vi "niFpga wdp fft pfft 8.vi"(6 "enable":bool, 11 "data in":T2(array[cluster])=[{"data re"=0.0, "data im"=0.0}, {"data re"=0.0, "data im"=0.0}, {"data re"=0.0, "data im"=0.0}, {"data re"=0.0, "data im"=0.0}, {"data re"=0.0, "data im"=0.0}, {"data re"=0.0, "data im"=0.0}, {"data re"=0.0, "data im"=0.0}, {"data re"=0.0, "data im"=0.0}]) -> (3 "data out":T1(array[cluster]))   [LabVIEW 2017]
uses:
  <vilib>/rvi/FXPMathLib/FxpSub/XNode/nifxpmath_Sub.xnode
  <vilib>/rvi/FXPMathLib/FxpAdd/XNode/nifxpmath_Add.xnode
  <vilib>/rvi/FXPMathLib/FxpMul/XNode/nifxpmath_Multiplier.xnode
  <vilib>/rvi/FXPMathLib/sim/FxpSim.dll
types:
  T1 = cluster{"data re":fxp<+/-,8,1>, "data re":fxp<+/-,8,1>}[]
  T2 = cluster{"data re":fxp<+/-,8,1>, "data im":fxp<+/-,8,1>}[]
  T3 = cluster{"data re":fxp<+/-,8,1>, "data im":fxp<+/-,8,1>}
  T4 = cluster{"data re":fxp<+/-,8,1>, "data re":fxp<+/-,8,1>}
  T5 = cluster{"x*y":fxp<+/-,25,4>, "x*y":fxp<+/-,25,4>}
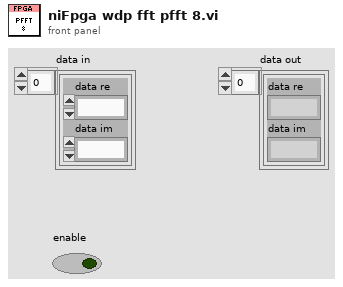
[diagram p1: front panel]
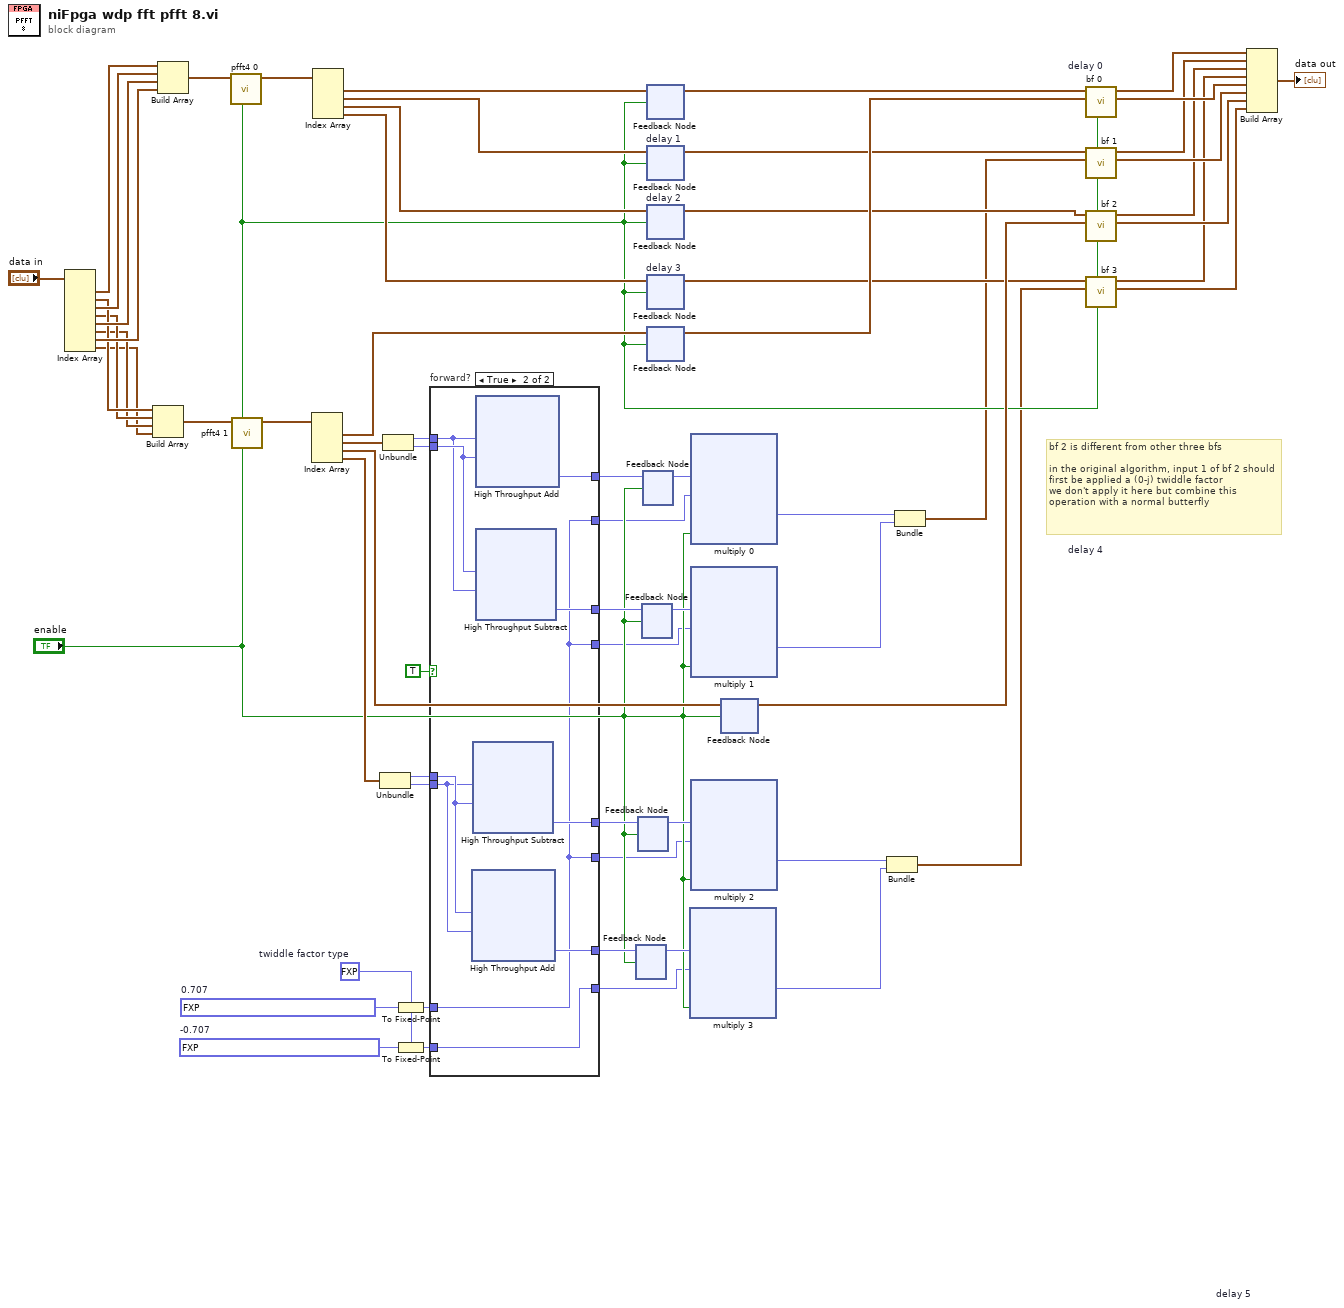
[diagram p0: block diagram]
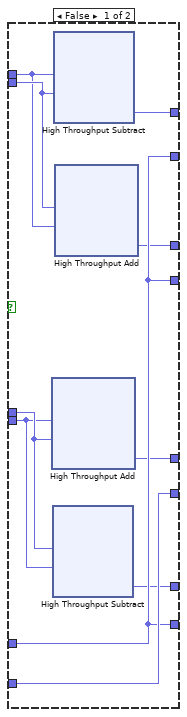
[diagram p2: hidden frame]
diagram:
  w36 = fxp<+/-,16,2> 0.0  # twiddle factor type
  w37 = fxp<+/-,32,2> -0.7071067811921239  # -0.707
  w38 = fxp<+/-,32,2> 0.7071067811921239  # 0.707
  # "bf 2 is different from other three bfs\n\nin the original algorithm, input 1 of bf 2 should first be applied a (0-j) twiddle factor\nwe don't apply it here but combine this operation with a normal butterfly"
  n1 = Index Array(array="data in") -> (element #1=w65:T3, element #2=w61:T3, element #3=w64:T3, element #4=w60:T3, element #5=w63:T3, element #6=w59:T3, element #7=w62:T3, element #8=w58:T3)  [unwired: 8 in]
  n2 = Build Array(w61, w60, w59, w58) -> (w32:T2)
  n3 = Build Array(w65, w64, w63, w62) -> (w34:T2)
  n4 = call "pfft4 0"("enable"="enable", "data in"=w34) -> ("data out"=w33:T1)  [unwired: 9 in]
  n5 = call "pfft4 1"("enable"="enable", "data in"=w32) -> ("data out"=w31:T1)  [unwired: 9 in]
  n6 = Index Array(array=w31) -> (element #1=w55:T4, element #2=w57:T4, element #3=w47:T4, element #4=w56:T4)  [unwired: 4 in]
  n7 = Index Array(array=w33) -> (element #1=w51:T4, element #2=w52:T4, element #3=w53:T4, element #4=w54:T4)  [unwired: 4 in]
  n8 = Unbundle(w56) -> ("data re"=w49:fxp<+/-,8,1>, "data re"=w48:fxp<+/-,8,1>)
  n9 = Unbundle(w57) -> ("data re"=w14:fxp<+/-,8,1>, "data re"=w50:fxp<+/-,8,1>)
  n10 = To Fixed-Point(fixed-point type=w36, number=w38) -> (fixed-point=w9:fxp<+/-,16,2>)
  n11 = To Fixed-Point(fixed-point type=w36, number=w37) -> (fixed-point=w7:fxp<+/-,16,2>)
  n12 = case "forward?" shown="True" TRUE {
    tunnel: w50 -> [w71 w85]
    tunnel: w49 -> [w68 w84]
    tunnel: w48 -> [w67 w83]
    tunnel: w14 -> [w70 w82]
    tunnel: [w73 w81] -> w46
    tunnel: [w72 w80] -> w44
    tunnel: [w69 w79] -> w42
    tunnel: [w66 w78] -> w40
    tunnel: [w74 w77] -> w12
    tunnel: [w74 w77] -> w11
    tunnel: [w75 w77] -> w10
    tunnel: w9 -> [w74 w77]
    tunnel: [w74 w76] -> w8
    tunnel: w7 -> [w75 w76]
    frame False {
      n13 = xnode ("High Throughput Add")("x"=w67, "y"=w68) -> ("x+y"=w69:fxp<+/-,9,2>)
      n14 = xnode "High Throughput Subtract"("x"=w68, "y"=w67) -> ("x-y"=w66:fxp<+/-,9,2>)
      n15 = xnode "High Throughput Subtract"("x"=w70, "y"=w71) -> ("x-y"=w73:fxp<+/-,9,2>)
      n16 = xnode ("High Throughput Add")("x"=w71, "y"=w70) -> ("x+y"=w72:fxp<+/-,9,2>)
    }
    frame True {
      n17 = xnode ("High Throughput Add")("x"=w84, "y"=w83) -> ("x+y"=w78:fxp<+/-,9,2>)
      n18 = xnode "High Throughput Subtract"("x"=w83, "y"=w84) -> ("x-y"=w79:fxp<+/-,9,2>)
      n19 = xnode ("High Throughput Add")("x"=w82, "y"=w85) -> ("x+y"=w81:fxp<+/-,9,2>)
      n20 = xnode "High Throughput Subtract"("x"=w85, "y"=w82) -> ("x-y"=w80:fxp<+/-,9,2>)
    }
  }
  n21 = feedback #1() -> (w39:fxp<+/-,9,2>)  [unwired: 1 in]
  n22 = feedback-in #1(w40, "enable") -> ()
  n23 = feedback #2() -> (w41:fxp<+/-,9,2>)  [unwired: 1 in]
  n24 = feedback-in #2(w42, "enable") -> ()
  n25 = feedback #3() -> (w43:fxp<+/-,9,2>)  [unwired: 1 in]
  n26 = feedback-in #3(w44, "enable") -> ()
  n27 = feedback #4() -> (w45:fxp<+/-,9,2>)  [unwired: 1 in]
  n28 = feedback-in #4(w46, "enable") -> ()
  n29 = feedback #5 "delay 0"() -> (w30:T4)  [unwired: 1 in]
  n30 = feedback-in #5(w51, "enable") -> ()
  n31 = feedback #6 "delay 1"() -> (w26:T4)  [unwired: 1 in]
  n32 = feedback-in #6(w52, "enable") -> ()
  n33 = feedback #7 "delay 2"() -> (w23:T4)  [unwired: 1 in]
  n34 = feedback-in #7(w53, "enable") -> ()
  n35 = feedback #8 "delay 3"() -> (w19:T4)  [unwired: 1 in]
  n36 = feedback-in #8(w54, "enable") -> ()
  n37 = feedback #9 "delay 4"() -> (w29:T4)  [unwired: 1 in]
  n38 = feedback-in #9(w55, "enable") -> ()
  n39 = xnode "multiply 3"("x"=w39, "y"=w8, "enable"="enable") -> ("x*y"=w5:fxp<+/-,25,4>)
  n40 = xnode "multiply 0"("x"=w45, "y"=w12, "enable"="enable") -> ("x*y"=w2:fxp<+/-,25,4>)
  n41 = xnode "multiply 1"("x"=w43, "y"=w11, "enable"="enable") -> ("x*y"=w3:fxp<+/-,25,4>)
  n42 = xnode "multiply 2"("x"=w41, "y"=w10, "enable"="enable") -> ("x*y"=w6:fxp<+/-,25,4>)
  n43 = feedback #10 "delay 5"() -> (w22:T4)  [unwired: 1 in]
  n44 = feedback-in #10(w47, "enable") -> ()
  n45 = Bundle("x*y"=w6, "x*y"=w5) -> (w4:T5)  [unwired: 1 in]
  n46 = Bundle("x*y"=w2, "x*y"=w3) -> (w1:T5)  [unwired: 1 in]
  n47 = call "bf 0"("enable"="enable", "data in 1"=w29, "data in 0"=w30) -> ("data out 1"=w27:T4, "data out 0"=w28:T4)  [unwired: 7 in]
  n48 = call "bf 1"("enable"="enable", "data in 1"=w1, "data in 0"=w26) -> ("data out 1"=w24:T4, "data out 0"=w25:T4)  [unwired: 7 in]
  n49 = call "bf 2"("enable"="enable", "data in 1"=w22, "data in 0"=w23) -> ("data out 1"=w21:T4, "data out 0"=w20:T4)  [unwired: 7 in]
  n50 = call "bf 3"("enable"="enable", "data in 1"=w4, "data in 0"=w19) -> ("data out 1"=w17:T4, "data out 0"=w18:T4)  [unwired: 7 in]
  n51 = Build Array(w28, w25, w20, w18, w27, w24, w21, w17) -> (→"data out":T1)
